vi "Create Waveform.vi"(8 "error in (no error)":errorcluster, 11 "Data1D in":refnum<class "Data1D.lvclass">) -> (0 "error out":errorcluster, 2 "Waveform":waveform(dbl), 3 "Data1D out":refnum<class "Data1D.lvclass">)   [LabVIEW 2014, in "Data1D.lvclass"]
uses:
  Data1D.lvclass
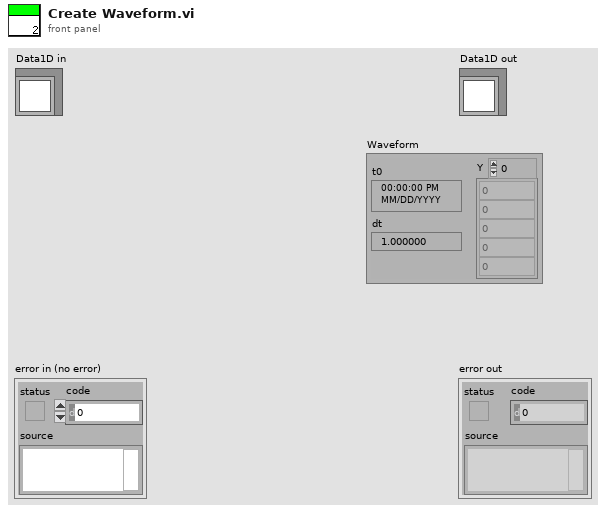
[diagram p1: front panel]
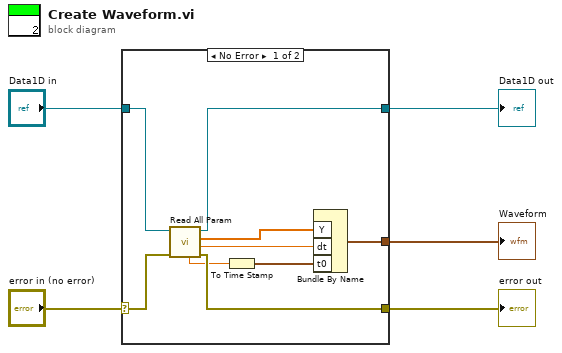
[diagram p0: block diagram]
diagram:
  n1 = case shown="No Error" "error in (no error)" {
    selector: "error in (no error)" -> [w10 w16]
    tunnel: [w9 w16] -> w4
    tunnel: [w11 w15] -> w2
    tunnel: "Data1D in" -> [w12 w15]
    tunnel: [w6 _] -> w1
    frame No Error {
      n2 = call "Read All Param.vi"("error in (no error)"=w10, "Data1D in"=w12) -> ("error out"=w9:errorcluster, "dt"=w13:dbl, "1D Array"=w14:dbl[], "Data1D out"=w11:refnum<class "Data1D.lvclass">, "t0"=w8:dbl)  [unwired: 5 in]
      n3 = To Time Stamp(1:w8) -> (0:w7:timestamp)
      n4 = Bundle By Name("Y"=w14, "dt"=w13, "t0"=w7) -> (w6:waveform(dbl))  [unwired: 1 in]
    }
    frame Error {
    }
  }
  "error out" <- w4
  "Data1D out" <- w2
  "Waveform" <- w1
